vi "OA_Controller_R.vi"(9 "Gait Phase":dbl, 10 "Weight":dbl, 11 "Walking Speed":dbl) -> (3 "Torque Output":dbl)   [LabVIEW 2019]
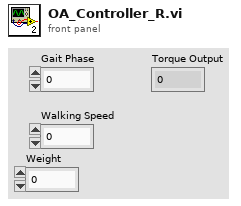
[diagram p1: front panel]
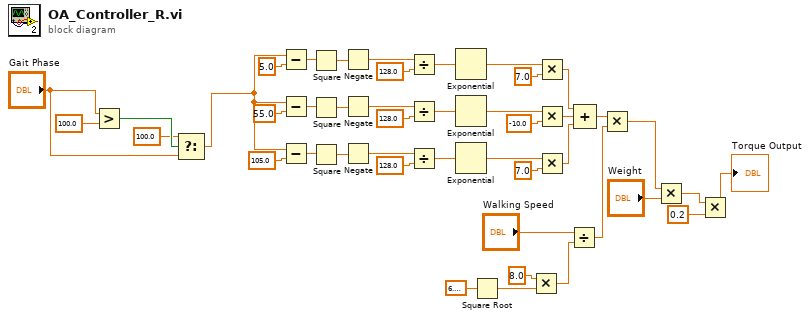
[diagram p0: block diagram]
diagram:
  n1 = Greater?(x="Gait Phase", y=100.0) -> (0:w4:bool)
  n2 = Select(t=100.0, s=w4, f="Gait Phase") -> (s? t:f=w1:dbl)
  n3 = Subtract(x=w1, y=5.0) -> (x-y=w11:dbl)
  n4 = Subtract(x=w1, y=55.0) -> (x-y=w19:dbl)
  n5 = Subtract(x=w1, y=105.0) -> (x-y=w27:dbl)
  n6 = Square(x=w11) -> (x^2=w12:dbl)
  n7 = Square(x=w19) -> (x^2=w20:dbl)
  n8 = Square(x=w27) -> (x^2=w28:dbl)
  n9 = Negate(x=w12) -> (-x=w13:dbl)
  n10 = Negate(x=w20) -> (-x=w21:dbl)
  n11 = Negate(x=w28) -> (-x=w29:dbl)
  n12 = Divide(x=w13, y=128.0) -> (x/y=w15:dbl)
  n13 = Divide(x=w21, y=128.0) -> (x/y=w23:dbl)
  n14 = Divide(x=w29, y=128.0) -> (x/y=w31:dbl)
  n15 = Exponential(1:w15) -> (0:w16:dbl)
  n16 = Exponential(1:w23) -> (0:w24:dbl)
  n17 = Exponential(1:w31) -> (0:w32:dbl)
  n18 = Square Root(x=6.283185307179586) -> (sqrt(x)=w43:dbl)
  n19 = Multiply(x=8.0, y=w43) -> (x*y=w41:dbl)
  n20 = Multiply(x=w16, y=7.0) -> (x*y=w35:dbl)
  n21 = Multiply(x=w24, y=-10.0) -> (x*y=w36:dbl)
  n22 = Multiply(x=w32, y=7.0) -> (x*y=w37:dbl)
  n23 = Divide(x="Walking Speed", y=w41) -> (x/y=w39:dbl)
  n24 = Compound Arithmetic op=ADD(w35, w36, w37) -> (w38:dbl)
  n25 = Multiply(x=w38, y=w39) -> (x*y=w10:dbl)
  n26 = Multiply(x=w10, y="Weight") -> (x*y=w8:dbl)
  n27 = Multiply(x=w8, y=0.2) -> (x*y=→"Torque Output":dbl)
